vi "getAllSubNodes.vi"(6 "filter Classes":string[](array[string]), 8 "error in (no error)":errorcluster, 10 "subNodes[]* in":refnum<data-value>[](array[refnum]), 11 "xceNode in":refnum<class "xceNode.lvclass">) -> (0 "error out":errorcluster, 2 "subNodes[]* out":refnum<data-value>[](array[refnum]), 3 "xceNode out":refnum<class "xceNode.lvclass">)   [LabVIEW 2013, in "xceNode.lvclass"]
doc: "Retrieves all nodes beneath this node, and returns their data value references. Use the option filter Classes input, you can restrict the type of classes that are returned."
uses:
  xceNode.lvclass
  xceTreeObj/xceTreeObj.lvclass
  xceNode.lvclass/xceNode.ctl
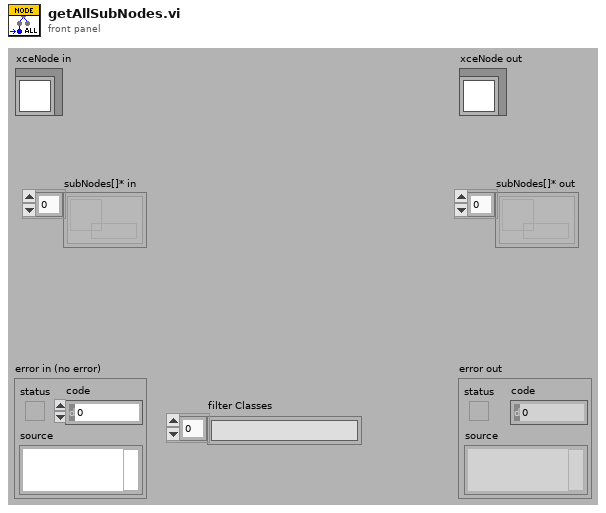
[diagram p1: front panel]
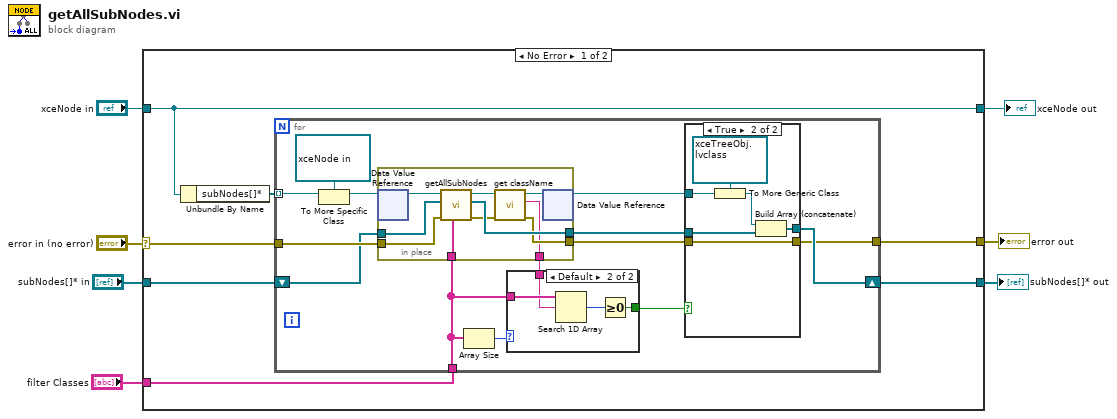
[diagram p0: block diagram]
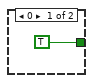
[diagram p3: hidden frame]
diagram:
  n1 = case shown="No Error" "error in (no error)" {
    selector: "error in (no error)" -> [w14 w53]
    tunnel: [w12 w53] -> w6
    tunnel: [w11 w52] -> w4
    tunnel: "xceNode in" -> [w11 w52]
    tunnel: "subNodes[]* in" -> [w9 _]
    tunnel: "filter Classes" -> [w13 _]
    tunnel: [w8 _] -> w1
    frame No Error {
      n2 = Unbundle By Name(w11) -> ("subNodes[]*"=w10:refnum<data-value>[])
      n3 = for {
        tunnel: w10 -> [w28] mode=indexing
        tunnel: w14 -> [w25]
        tunnel: [w15] -> w12
        tunnel: w13 -> [w19]
        shift-right: [w21] -> w8
        shift-left: w9 -> [w22]
        n4 = To More Specific Class(target class=refnum<data-value> refnum ("data value reference"), reference=w28) -> (specific class reference=w26:refnum<data-value>)  [unwired: 1 in, 1 out]
        n5 = in-place {
          in-place-border: w25 -> [w50]
          in-place-border: [w43] -> w16
          in-place-border: w19 -> [w49]
          in-place-border: [w48] -> w24
          in-place-border: w22 -> [w47]
          in-place-border: [w42] -> w20
          n6 = in-place-dvr #1(w26) -> (w51:refnum<class "xceNode.lvclass">)  [unwired: 1 out]
          n7 = call "getAllSubNodes.vi"("filter Classes"=w49, "error in (no error)"=w50, "subNodes[]* in"=w47, "xceNode in"=w51) -> ("error out"=w44:errorcluster, "subNodes[]* out"=w48:refnum<data-value>[], "xceNode out"=w46:refnum<class "xceNode.lvclass">)  [unwired: 5 in]
          n8 = call "get className.vi"("error in (no error)"=w44, "xceNode in"=w46) -> ("error out"=w43:errorcluster, "Class name"=w42:string, "xceNode out"=w45:refnum<class "xceNode.lvclass">)  [unwired: 7 in]
          n9 = in-place-dvr #1(w45) -> (w23:refnum<data-value>)  [unwired: 1 out]
        }
        n10 = Array Size(array=w19) -> (size(s)=w18:i32)
        n11 = case shown="Default" w18 {
          tunnel: w19 -> [_ w41]
          tunnel: w20 -> [_ w40]
          tunnel: [TRUE w39] -> w17
          frame 0 {
          }
          frame Default {
            n12 = Search 1D Array(1D array=w41, element=w40) -> (index of element=w38:i32)  [unwired: 1 in]
            n13 = Greater Or Equal To 0?(x=w38) -> (x >= 0?=w39:bool)
          }
        }
        n14 = case shown="True" w17 {
          tunnel: w24 -> [w30 w36]
          tunnel: w23 -> [_ w35]
          tunnel: [w30 w32] -> w21
          tunnel: w16 -> [w29 w31]
          tunnel: [w29 w31] -> w15
          frame False {
          }
          frame True {
            n15 = To More Generic Class(target class=refnum<data-value> refnum ("superNode*"), reference=w35) -> (generic class reference=w33:refnum<data-value>)
            n16 = Build Array (concatenate)(w33, w36) -> (w32:refnum<data-value>[])
          }
        }
      }
    }
    frame Error {
    }
  }
  "error out" <- w6
  "xceNode out" <- w4
  "subNodes[]* out" <- w1
